vi "UI_AutoRefresh_Init.vi"(8 "error in (no error)":errorcluster, 10 "Parameters":T1={"Write TipStrips with details (T)"=TRUE, "Write Captions with UserLabels (T)"=TRUE, "Mode (ind only)"=enum."Indicators only", "Enable nested stream (T)"=TRUE}, 11 "SingleIndi in":refnum<class "SingleIndi.lvclass">) -> (0 "error out":errorcluster, 3 "SingleIndi out":refnum<class "SingleIndi.lvclass">)   [LabVIEW 2020, in "SingleIndi.lvlib" / "SingleIndi.lvclass"]
uses:
  SingleIndi.lvclass
  D:/Projets/IRSN/464 - IRSN - LEF/464-irsn-lef-hmi/support/UI_Actor.lvlibp/UI_Actor/UI_Actor.lvclass
  support/UI_Actor.lvlibp/UI_Actor/ctl_AR_Parameters.ctl
  support/UI_Actor.lvlibp/UI_Actor/ctl_AR_Mode.ctl
  support/Databox.lvlibp/TypesTools/Config/Read System Label.vi
  support/Databox.lvlibp/TypesTools/Config/Read User Label.vi
  support/UI_Actor.lvlibp/UI_Actor/UI_Elmt_Ref(Label).vi
  D&C_SchemaBase/D&C_SchemaBase/D&C_SchemaBase.lvclass
  support/UI_Actor.lvlibp/UI_Actor/UI_Actor.lvclass
  D:/Projets/IRSN/464 - IRSN - LEF/464-irsn-lef-hmi/D&Cs/D&C_SchemaBase/D&C_SchemaBase/D&C_SchemaBase.lvclass
  D:/Projets/IRSN/464 - IRSN - LEF/464-irsn-lef-hmi/support/Actor Framework.lvlibp/1abvi3w/vi.lib/ActorFramework/Actor/Actor.lvclass
  D:/Projets/IRSN/464 - IRSN - LEF/464-irsn-lef-hmi/D&Cs/SingleIndi/SingleIndi/SingleIndi.lvclass
  support/Databox.lvlibp/TypesTools/Config/Config.lvclass
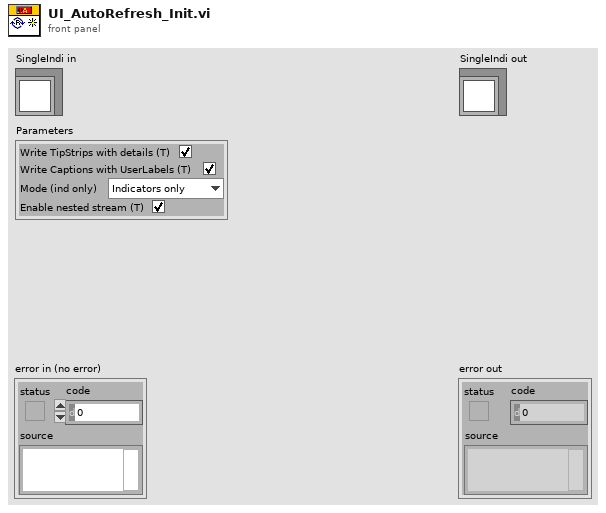
[diagram p1: front panel]
types:
  T1 = typedef "UI_Actor.lvlibp/UI_Actor.lvclass/ctl_AR_Parameters.ctl" = cluster{"Write TipStrips with details (T)":bool, "Write Captions with UserLabels (T)":bool, "Mode (ind only)":T2, "Enable nested stream (T)":bool}
  T2 = typedef "UI_Actor.lvlibp/UI_Actor.lvclass/ctl_AR_Mode.ctl" = enum16{"Controls only", "Indicators only", "All"}
  T3 = typedef "UI_Actor.lvlibp/UI_Actor.lvclass/ctl_InternalMapItem.ctl" = cluster{"Config":refnum<class "Config.lvclass">, "LatestData":refnum<class "Data.lvclass">}
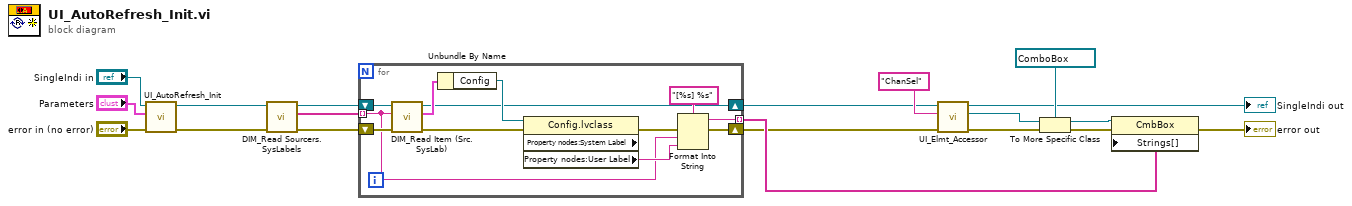
[diagram p0: block diagram]
diagram:
  n1 = call-parent "UI_AutoRefresh_Init.vi"("error in (no error)"="error in (no error)", "Parameters"="Parameters", "UI_Actor in"="SingleIndi in") -> ("error out"=w15:errorcluster, "UI_Actor out"=w16:refnum<class "SingleIndi.lvclass">)  [unwired: 7 in]
  n2 = call "DIM_Read Sourcers.SysLabels.vi"("error in (no error)"=w15, "UI_Actor in"=w16) -> ("error out"=w2:errorcluster, "DIM Sourcer.SysLabels"=w5:string[], "UI_Actor out"=w6:refnum<class "SingleIndi.lvclass">)  [unwired: 7 in]
  n3 = for {
    tunnel: w5 -> [w20] mode=indexing
    tunnel: [w24] -> w4 mode=indexing
    shift-right: [w23] -> w3
    shift-left: w2 -> [w22]
    shift-right: [w21] -> w1
    shift-left: w6 -> [w25]
    n4 = call "DIM_Read Item (Src.SysLab).vi"("error in (no error)"=w22, "Sourcer.SysLabel"=w20, "UI_Actor in"=w25) -> ("error out"=w27:errorcluster, "DIM Item"=w31:T3, "UI_Actor out"=w21:refnum<class "SingleIndi.lvclass">)  [unwired: 5 in, 1 out]
    n5 = Unbundle By Name(w31) -> ("Config"=w30:refnum<class "Config.lvclass">)
    n6 = property class="Config.lvclass" props=["Property nodes:System Label", "Property nodes:User Label"](reference=w30, error in=w27) -> (error out=w26:errorcluster, "Property nodes:User Label"=w28:string)  [unwired: 2 out]
    n7 = Format Into String(format string="[%s] %s", error in=w26, w20, w28) -> (resulting string=w24:string, error out=w23:errorcluster)  [unwired: 1 in]
  }
  n8 = call-poly "UI_Elmt_Accessor.vi"("error in (no error)"=w3, "Elmt Label"="ChanSel", "UI_Actor in"=w1) -> ("error out"=w10:errorcluster, "Ctl Refnum"=w11:refnum<vi>, "UI_Actor out"=→"SingleIndi out":refnum<class "SingleIndi.lvclass">)  [unwired: 5 in, 1 out]
  n9 = To More Specific Class(target class=refnum<vi> refnum ("ChanSel"), reference=w11, error in=w10) -> (specific class reference=w9:refnum<vi>, error out=w8:errorcluster)
  n10 = property class="CmbBox"(reference=w9, error in=w8, "Strings[]"=w4) -> (error out=→"error out":errorcluster)  [unwired: 1 out]
